vi "Create Loaded Stat Bundle.vi"(7 "StatArray":string[][](array[string]), 11 "CMD Step":dbl format="%#_13g") -> (8 "StatBundle Out":T1(array[cluster]))   [LabVIEW 2013]
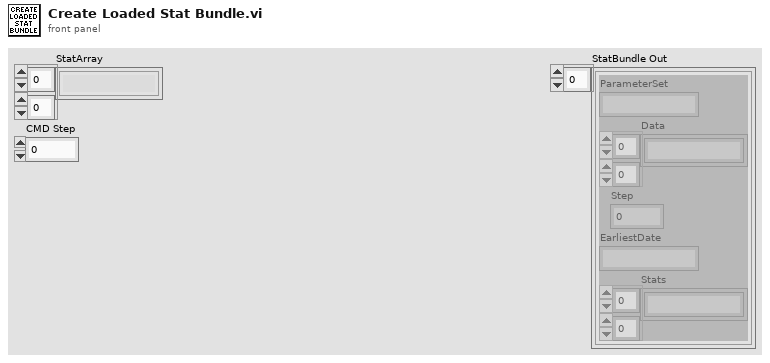
[diagram p1: front panel]
types:
  T1 = cluster{"ParameterSet":string, "Data":string[][], "Step":i32, "EarliestDate":string, "Stats":string[][]}[]
  T2 = typedef "Command Cluster.ctl" = cluster{"Para1":i32, "SP1":dbl, "Para2":i32, "SP2":dbl, "Para3":i32, "SP3":dbl}
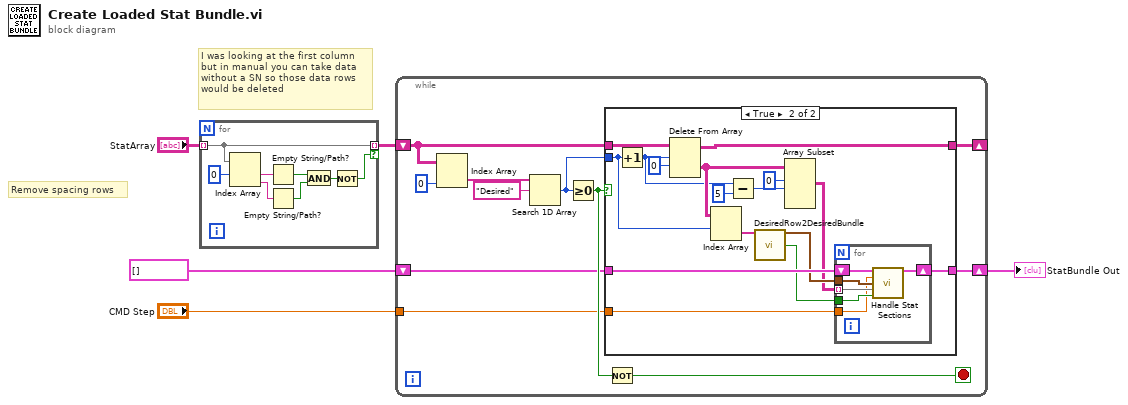
[diagram p0: block diagram]
diagram:
  # "I was looking at the first column\nbut in manual you can take data\nwithout a SN so those data rows\nwould be deleted"
  # "Remove spacing rows"
  n1 = for {
    tunnel: "StatArray" -> [w11] mode=indexing
    tunnel: [w11] -> w4 mode=indexing if=w10
    n2 = Index Array(array=w11, index #1=0 ("index")) -> (element #1=w12:string, element #2=w9:string)  [unwired: 1 in]
    n3 = Empty String/Path?(string/path=w12) -> (empty?=w8:bool)
    n4 = Empty String/Path?(string/path=w9) -> (empty?=w7:bool)
    n5 = And(x=w8, y=w7) -> (x .and. y?=w6:bool)
    n6 = Not(x=w6) -> (.not. x?=w10:bool)
  }
  n7 = while {
    shift-right: [w20] -> _
    shift-left: w4 -> [w21]
    shift-right: [w16] -> w2
    shift-left: T1 [] ("StatBundle") -> [w17]
    tunnel: "CMD Step" -> [w14]
    stop <- w18 stop-if-true
    n8 = Index Array(array=w21, index (col)=0 ("disabled index (col)")) -> (element=w23:string[])  [unwired: 1 in]
    n9 = Search 1D Array(1D array=w23, element="Desired") -> (index of element=w15:i32)  [unwired: 1 in]
    n10 = Greater Or Equal To 0?(x=w15) -> (x >= 0?=w19:bool)
    n11 = case shown="True" w19 {
      tunnel: w21 -> [w26 w42]
      tunnel: w15 -> [_ w35]
      tunnel: [w26 w40] -> w20
      tunnel: w17 -> [w25 w38]
      tunnel: [w25 w39] -> w16
      tunnel: w14 -> [_ w27]
      frame False {
      }
      frame True {
        n12 = Increment(x=w35) -> (x+1=w31:i32)
        n13 = Delete From Array(array=w42, length=w31, index (row)=0) -> (deleted portion=w33:string[][], array with subset deleted=w40:string[][])  [unwired: 1 in]
        n14 = Index Array(array=w33, index (row)=w35) -> (element=w34:string[])  [unwired: 1 in]
        n15 = Subtract(x=w31, y=5) -> (x-y=w30:i32)
        n16 = call "DesiredRow2DesiredBundle.vi"("DesiredStatRow"=w34) -> ("DesiredParameters"=w36:T2, "Controller?"=w37:bool)  [unwired: 13 in]
        n17 = Array Subset(array=w33, index (row)=0 ("index"), length (row)=w30) -> (w28:string[][])  [unwired: 2 in]
        n18 = for {
          shift-right: [w48] -> w39
          shift-left: w38 -> [w47]
          tunnel: w28 -> [w46] mode=indexing
          tunnel: w37 -> [w45]
          tunnel: w36 -> [w44]
          tunnel: w27 -> [w43]
          n19 = call "Handle Stat Sections.vi"("StatBundle In"=w47, "CMD Step"=w43, "DesiredParameters"=w44, "LastDataSet"=w46, "Controller?"=w45) -> ("StatBundle Out"=w48:T1)  [unwired: 10 in]
        }
      }
    }
    n20 = Not(x=w19) -> (.not. x?=w18:bool)
  }
  "StatBundle Out" <- w2
